vi "Test Gauge Ramp Alarm.vi"() -> ()   [LabVIEW 2012]
uses:
  Controls/Gauge TDef.ctl
  Controls/Alarm Limits TDef.ctl
panel:
  in  "Hi Alarm":T1={"Flow"=0.0, "Fuel Temp"=350.0, "Supply Pressure"=100.0, "Diff. Pressure (50psid)"=100.0, "Back Pressure"=100.0, "Bypass Pressure"=100.0, "Diff. Pressure (100psid)"=100.0, "BP (Monitor)"=0.0}
  in  "LoAlarm":T1={"Flow"=0.0, "Fuel Temp"=0.0, "Supply Pressure"=20.0, "Diff. Pressure (50psid)"=20.0, "Back Pressure"=20.0, "Bypass Pressure"=20.0, "Diff. Pressure (100psid)"=20.0, "BP (Monitor)"=0.0}
  in  "Current Flow Limits":cluster{"Low Limit":dbl, "Hi Limit":dbl}
  in  "Analog Sensors":T2 {"Fuel Temp" scale=0.0..100.0; "Flow" scale=0.01..2.0; "Unused" scale=0.0..10.0; "Diff. Pressure (100psid)" scale=0.0..10.0; "Bypass Pressure" scale=0.0..60.0; "Back Pressure" scale=0.0..10.0; "Diff. Pressure  (50 psid)" scale=0.0..10.0; "Supply Pressure" scale=0.0..3000.0}
  in  "stop":bool
  out "Analog Sensors":T2 {"Fuel Temp" scale=0.0..100.0; "Flow" scale=0.0..5000.0; "Unused" scale=0.0..20.0; "Diff. Pressure (100psid)" scale=0.0..100.0; "Bypass Pressure" scale=0.0..100.0; "Back Pressure" scale=0.0..100.0; "Diff. Pressure  (50 psid)" scale=0.0..100.0; "Supply Pressure" scale=0.0..1000.0}
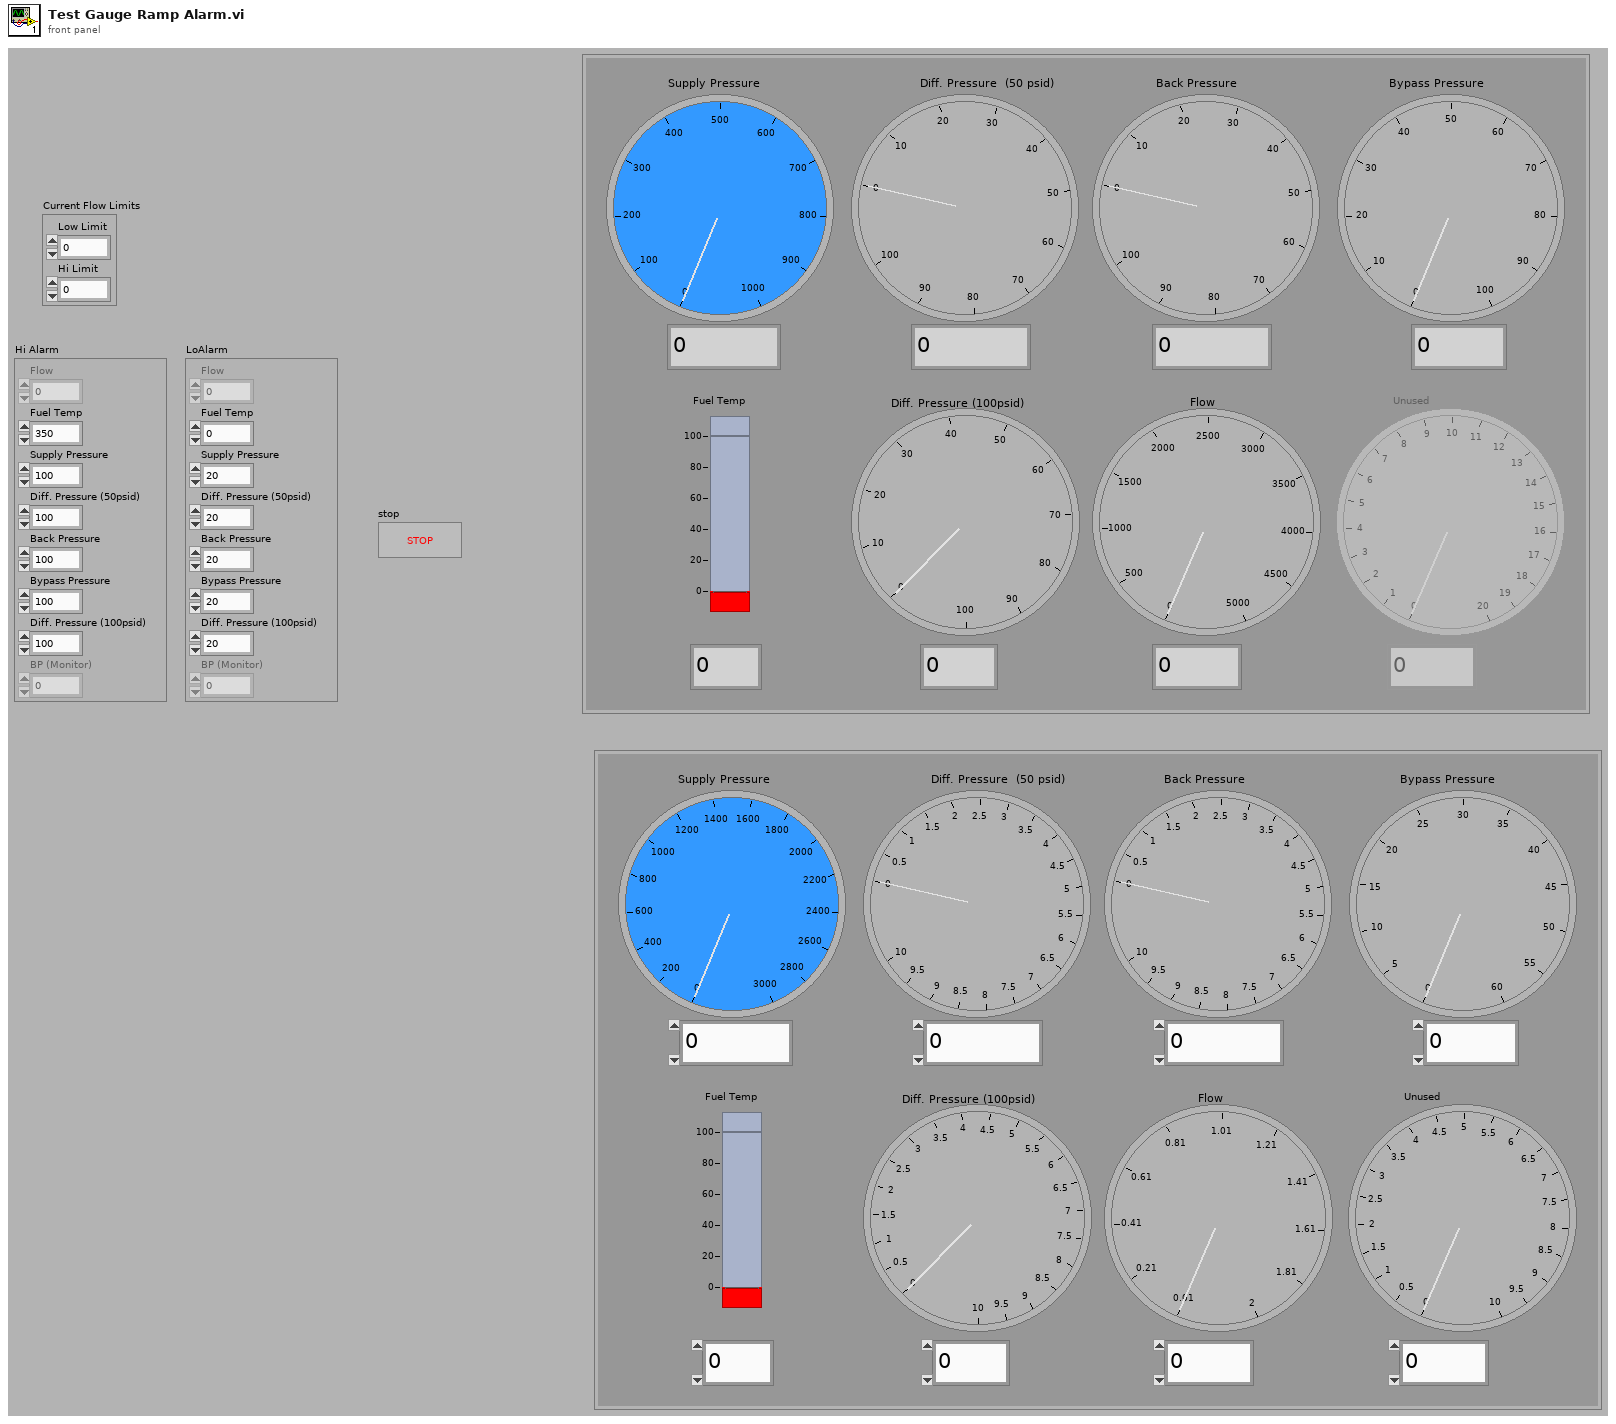
[diagram p1: front panel]
types:
  T1 = typedef "Alarm Limits TDef.ctl" = cluster{"Flow":dbl, "Fuel Temp":dbl, "Supply Pressure":dbl, "Diff. Pressure (50psid)":dbl, "Back Pressure":dbl, "Bypass Pressure":dbl, "Diff. Pressure (100psid)":dbl, "BP (Monitor)":dbl}
  T2 = typedef "Gauge TDef.ctl" = cluster{"Flow":dbl, "Fuel Temp":dbl, "Supply Pressure":dbl, "Diff. Pressure  (50 psid)":dbl, "Back Pressure":dbl, "Bypass Pressure":dbl, "Diff. Pressure (100psid)":dbl, "Unused":dbl}
  T3 = enum16{"Init", "Add Alarm Limits", "Update Flow Limit", "Check for Alarm", "Clear Alarms"}
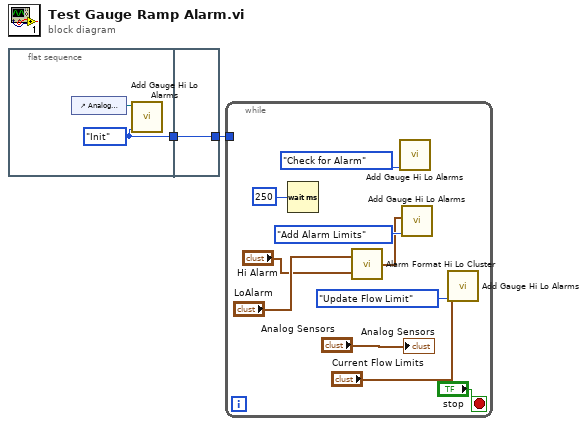
[diagram p0: block diagram]
diagram:
  n1 = flat-sequence {
    tunnel: [w3] -> w1
    tunnel: [w5] -> w2
    tunnel: w1 -> [w5]
    frame #0 {
      w3 = T3."Init" ("Action")
      n2 = control-ref of="Analog Sensors"() -> (w4:refnum<vi>)
      n3 = call "Add Gauge Hi Lo Alarms.vi"("Action"=w3, "reference"=w4) -> ()  [unwired: 9 in]
    }
    frame #1 {
    }
  }
  n4 = while {
    tunnel: w2 -> [_]
    stop <- "stop" stop-if-true
    n5 = Wait (ms)(milliseconds to wait=u32 250) -> ()  [unwired: 1 out]
    n6 = call "Alarm Format Hi Lo Cluster.vi"("HI Alarm"="Hi Alarm", "LO Alarm"="LoAlarm") -> ("Limits"=w8:cluster{"Lo":dbl, "Hi":dbl}[])
    n7 = call "Add Gauge Hi Lo Alarms.vi"("Action"=T3."Check for Alarm") -> ()  [unwired: 10 in]
    n8 = call "Add Gauge Hi Lo Alarms.vi"("Action"=T3."Add Alarm Limits", "Limits"=w8) -> ()  [unwired: 9 in]
    n9 = call "Add Gauge Hi Lo Alarms.vi"("Action"=T3."Update Flow Limit", "Current Flow Limits"="Current Flow Limits") -> ()  [unwired: 9 in]
    "Analog Sensors" <- "Analog Sensors"
  }
